vi "Projectile Trajectory Graph.vi"(6 "X Velocity":dbl, 7 "Initial Height":dbl, 9 "Gravitational Acceleration":dbl, 10 "Initial Y Velocity":dbl, 11 "End Time":dbl) -> (3 "Trajectory Graph":cluster{"Y Values":dbl[], "Y Values":dbl[]}(graph))   [LabVIEW 2016]
uses:
  <vilib>/gmath/NI_Gmath.lvlib
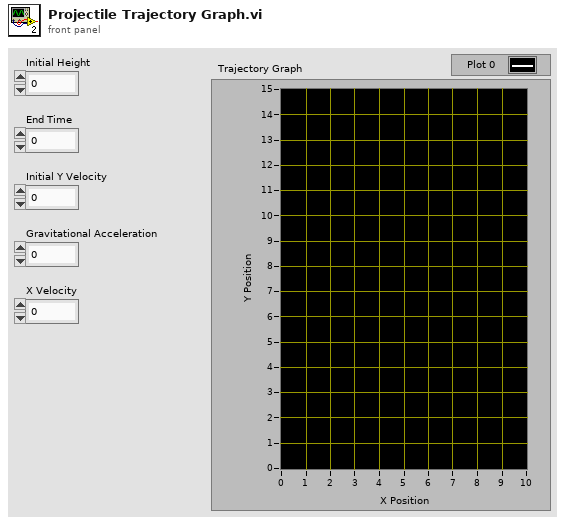
[diagram p1: front panel]
types:
  T1 = cluster{"parameter name":string, "parameter content":string}
  T2 = cluster{"parameter name":string, "parameter content":string}[]
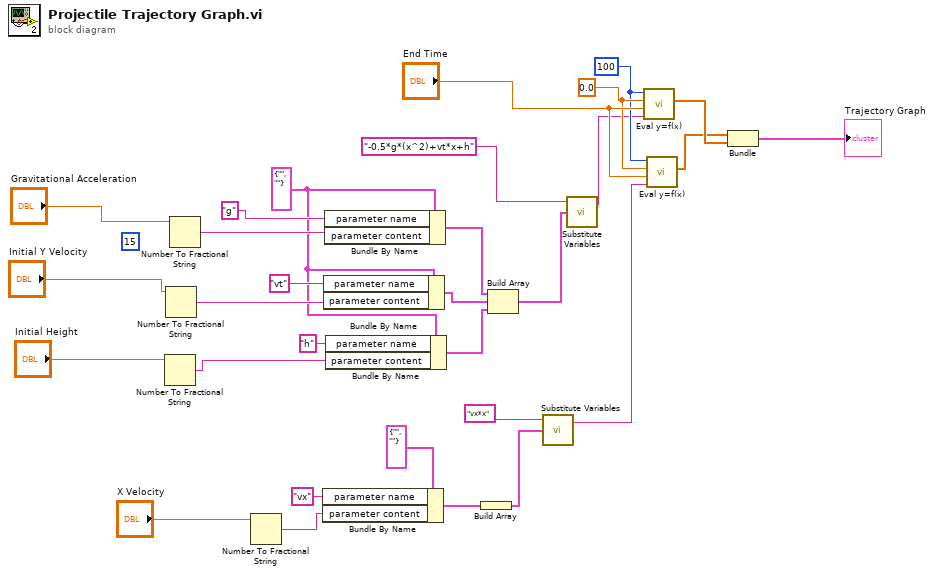
[diagram p0: block diagram]
diagram:
  (unwired) i16 15 ("width (-)")
  w3 = T1 {"parameter name"="", "parameter content"=""}
  w24 = u32 100 ("number of points")
  w25 = 0.0 ("start")
  n1 = Number To Fractional String(number="Initial Height") -> (F-format string=w12:string)  [unwired: 3 in]
  n2 = Number To Fractional String(number="Initial Y Velocity") -> (F-format string=w11:string)  [unwired: 3 in]
  n3 = Number To Fractional String(number="Gravitational Acceleration") -> (F-format string=w8:string)  [unwired: 3 in]
  n4 = Number To Fractional String(number="X Velocity") -> (F-format string=w22:string)  [unwired: 3 in]
  n5 = Bundle By Name(cluster=T1 {"parameter name"="", "parameter content"=""}, "parameter name"="vx", "parameter content"=w22) -> (w19:T1)
  n6 = Bundle By Name(cluster=w3, "parameter name"="vt", "parameter content"=w11) -> (w4:T1)
  n7 = Bundle By Name(cluster=w3, "parameter name"="g", "parameter content"=w8) -> (w2:T1)
  n8 = Bundle By Name(cluster=w3, "parameter name"="h", "parameter content"=w12) -> (w5:T1)
  n9 = Build Array(w19) -> (w20:T2)
  n10 = Build Array(w2, w4, w5) -> (w6:T2)
  n11 = call <vilib>:"Substitute Variables.vi"("Substitution Rules"=w20, "original formula"="vx*x") -> ("formula after substitution"=w26:string)  [unwired: 1 in, 1 out]
  n12 = call <vilib>:"Substitute Variables.vi"("Substitution Rules"=w6, "original formula"="-0.5*g*(x^2)+vt*x+h") -> ("formula after substitution"=w9:string)  [unwired: 1 in, 1 out]
  n13 = call <vilib>:"Eval y=f(x).vi"("formula"=w9, "end"="End Time", "start"=w25, "number of points"=w24) -> ("Y Values"=w29:dbl[])  [unwired: 3 out]
  n14 = call <vilib>:"Eval y=f(x).vi"("formula"=w26, "end"="End Time", "start"=w25, "number of points"=w24) -> ("Y Values"=w28:dbl[])  [unwired: 3 out]
  n15 = Bundle("Y Values"=w28, "Y Values"=w29) -> (→"Trajectory Graph":cluster{"Y Values":dbl[], "Y Values":dbl[]})  [unwired: 1 in]
